vi "encoder distance calc.vi"(8 "BR":dbl, 9 "BL":dbl, 10 "FR":dbl, 11 "FL":dbl) -> (1 "twist":dbl, 2 "X":dbl, 3 "Y":dbl)   [LabVIEW 2012]
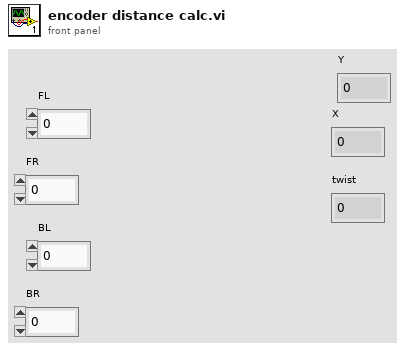
[diagram p1: front panel]
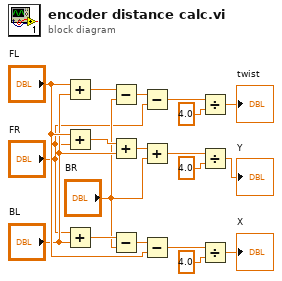
[diagram p0: block diagram]
diagram:
  n1 = Add(x="FL", y="BL") -> (x+y=w5:dbl)
  n2 = Add(x="FL", y="FR") -> (x+y=w17:dbl)
  n3 = Add(x="FR", y="BL") -> (x+y=w10:dbl)
  n4 = Subtract(x=w5, y="BR") -> (x-y=w4:dbl)
  n5 = Add(x=w17, y="BL") -> (x+y=w16:dbl)
  n6 = Subtract(x=w10, y="BR") -> (x-y=w9:dbl)
  n7 = Subtract(x=w4, y="FR") -> (x-y=w3:dbl)
  n8 = Add(x=w16, y="BR") -> (x+y=w15:dbl)
  n9 = Subtract(x=w9, y="FL") -> (x-y=w8:dbl)
  n10 = Divide(x=w3, y=4.0) -> (x/y=→"twist":dbl)
  n11 = Divide(x=w15, y=4.0) -> (x/y=→"Y":dbl)
  n12 = Divide(x=w8, y=4.0) -> (x/y=→"X":dbl)
